vi "Lab 3 - Monty Hall.vi"() -> ()   [LabVIEW 2025]
panel:
  in  "Door 3":bool
  in  "Door 2":bool
  in  "Door 1":bool
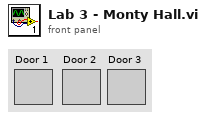
[diagram p1: front panel]
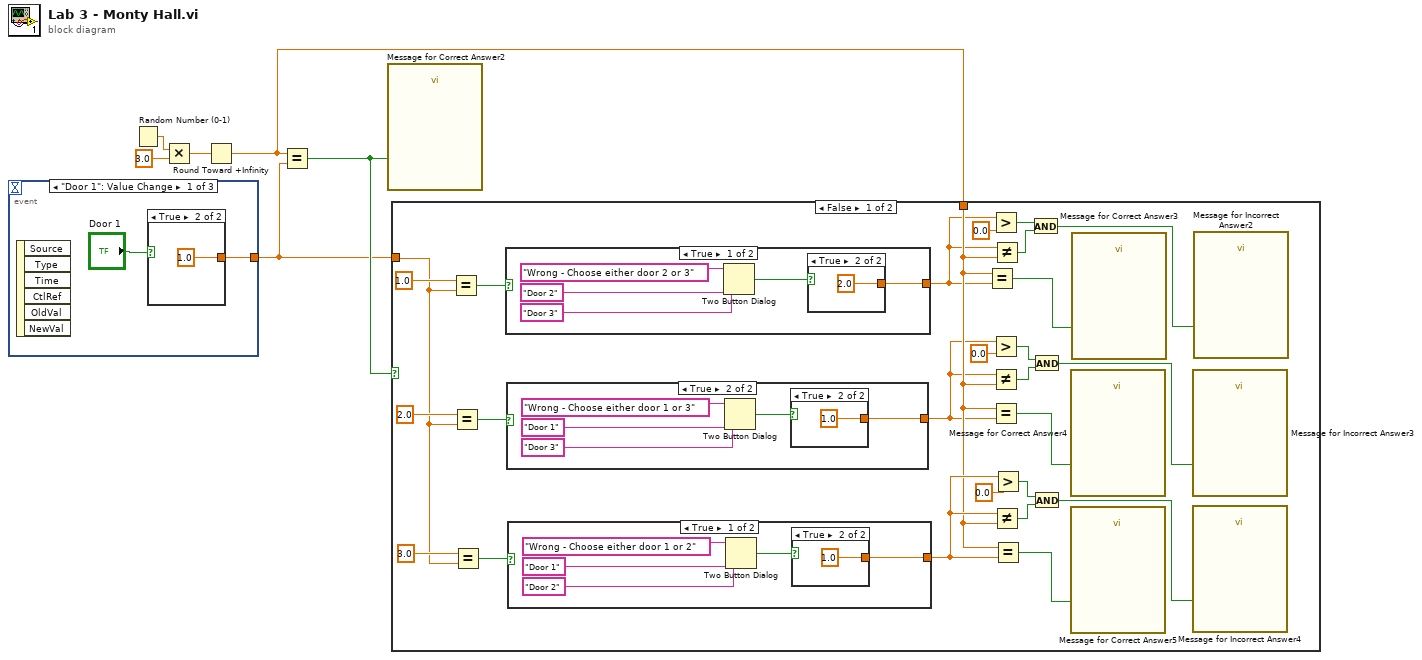
[diagram p0: block diagram]
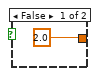
[diagram p2: hidden frame]
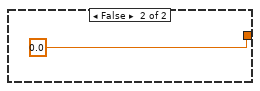
[diagram p3: hidden frame]
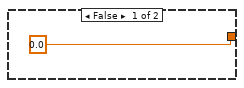
[diagram p4: hidden frame]
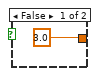
[diagram p5: hidden frame]
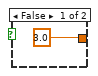
[diagram p6: hidden frame]
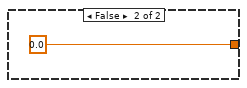
[diagram p7: hidden frame]
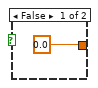
[diagram p9: hidden frame]
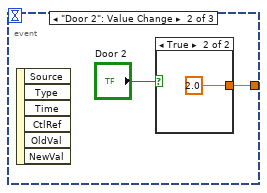
[diagram p10: hidden frame]
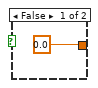
[diagram p11: hidden frame]
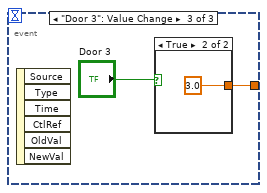
[diagram p12: hidden frame]
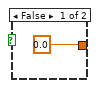
[diagram p13: hidden frame]
diagram:
  n1 = event shown="[0] \"Door 1\": Value Change" {
    selector: _ -> [_ _ _]
    dyn-events: _ -> [_ _ _]
    timeout: _ -> [_ _ _]
    tunnel: [w7 w11 w15] -> w3
    event "Door 1": Value Change {
      n2 = event-data() -> ()  [unwired: 1 in, 6 out]
      n3 = case shown="True" "Door 1" {
        tunnel: [0.0 1.0] -> w7
        frame False {
        }
        frame True {
        }
      }
    }
    event "Door 2": Value Change {
      n4 = event-data() -> ()  [unwired: 1 in, 6 out]
      n5 = case shown="True" "Door 2" {
        tunnel: [0.0 2.0] -> w11
        frame False {
        }
        frame True {
        }
      }
    }
    event "Door 3": Value Change {
      n6 = event-data() -> ()  [unwired: 1 in, 6 out]
      n7 = case shown="True" "Door 3" {
        tunnel: [0.0 3.0] -> w15
        frame False {
        }
        frame True {
        }
      }
    }
  }
  n8 = Random Number (0-1)() -> (number: 0 to 1=w5:dbl)
  n9 = Multiply(x=w5, y=3.0) -> (x*y=w2:dbl)
  n10 = Round Toward +Infinity(x=w2) -> (ceil(x): smallest int >= x=w1:dbl)
  n11 = Equal?(x=w1, y=w3) -> (x = y?=w4:bool)
  n12 = call "Message for Correct Answer2"("Enable"=w4) -> ()  [unwired: 9 in, 2 out]
  n13 = case shown="False" w4 {
    tunnel: w3 -> [w38 _]
    tunnel: w1 -> [w25 _]
    frame False {
      n14 = Equal?(x=1.0, y=w38) -> (x = y?=w41:bool)
      n15 = Equal?(x=2.0, y=w38) -> (x = y?=w39:bool)
      n16 = Equal?(x=3.0, y=w38) -> (x = y?=w40:bool)
      n17 = case shown="True" w41 {
        tunnel: [w61 0.0] -> w24
        frame True {
          n18 = Two Button Dialog(message="Wrong - Choose either door 2 or 3", 1:"Door 3", 2:"Door 2") -> (T button?=w62:bool)
          n19 = case shown="True" w62 {
            tunnel: [3.0 2.0] -> w61
            frame False {
            }
            frame True {
            }
          }
        }
        frame False {
        }
      }
      n20 = case shown="True" w39 {
        tunnel: [0.0 w54] -> w23
        frame False {
        }
        frame True {
          n21 = Two Button Dialog(message="Wrong - Choose either door 1 or 3", 1:"Door 3", 2:"Door 1") -> (T button?=w55:bool)
          n22 = case shown="True" w55 {
            tunnel: [3.0 1.0] -> w54
            frame False {
            }
            frame True {
            }
          }
        }
      }
      n23 = case shown="True" w40 {
        tunnel: [w45 0.0] -> w28
        frame True {
          n24 = Two Button Dialog(message="Wrong - Choose either door 1 or 2", 1:"Door 2", 2:"Door 1") -> (T button?=w46:bool)
          n25 = case shown="True" w46 {
            tunnel: [2.0 1.0] -> w45
            frame False {
            }
            frame True {
            }
          }
        }
        frame False {
        }
      }
      n26 = Equal?(x=w25, y=w24) -> (x = y?=w37:bool)
      n27 = Greater?(x=w24, y=0.0) -> (0:w21:bool)
      n28 = Greater?(x=w23, y=0.0) -> (0:w26:bool)
      n29 = Not Equal?(x=w23, y=w25) -> (x != y?=w27:bool)
      n30 = Equal?(x=w25, y=w23) -> (x = y?=w36:bool)
      n31 = Not Equal?(x=w24, y=w25) -> (x != y?=w22:bool)
      n32 = Not Equal?(x=w28, y=w25) -> (x != y?=w29:bool)
      n33 = Greater?(x=w28, y=0.0) -> (0:w31:bool)
      n34 = Equal?(x=w25, y=w28) -> (x = y?=w35:bool)
      n35 = And(x=w21, y=w22) -> (x .and. y?=w20:bool)
      n36 = And(x=w26, y=w27) -> (x .and. y?=w19:bool)
      n37 = And(x=w31, y=w29) -> (x .and. y?=w30:bool)
      n38 = call "Message for Correct Answer4"("Enable"=w36) -> ()  [unwired: 9 in, 2 out]
      n39 = call "Message for Correct Answer5"("Enable"=w35) -> ()  [unwired: 9 in, 2 out]
      n40 = call "Message for Correct Answer3"("Enable"=w37) -> ()  [unwired: 9 in, 2 out]
      n41 = call "Message for Incorrect Answer3"("Enable"=w19) -> ()  [unwired: 9 in, 2 out]
      n42 = call "Message for Incorrect Answer4"("Enable"=w30) -> ()  [unwired: 9 in, 2 out]
      n43 = call "Message for Incorrect Answer2"("Enable"=w20) -> ()  [unwired: 9 in, 2 out]
    }
    frame True {
    }
  }
